vi "Get Input Index.vi"(8 "error in (no error)":errorcluster, 10 "Input Name":string, 11 "Mux in":refnum<class "Mux.lvclass">) -> (0 "error out":errorcluster, 1 "Found?":bool, 2 "Input Index":i32, 3 "Mux out":refnum<class "Mux.lvclass">)   [LabVIEW 2022 SP3]
uses:
  Mux.lvclass
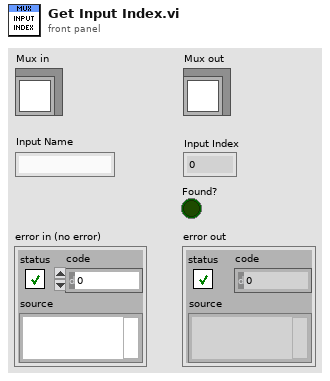
[diagram p1: front panel]
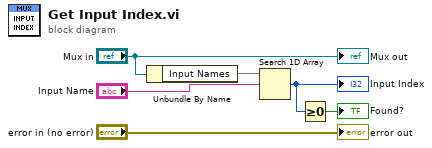
[diagram p0: block diagram]
diagram:
  n1 = Unbundle By Name("Mux in") -> ("Input Names"=w4)
  n2 = Search 1D Array(1D array=w4, element="Input Name") -> (index of element=w2:i32)  [unwired: 1 in]
  "Input Index" <- w2
  n3 = Greater Or Equal To 0?(x=w2) -> (x >= 0?=→"Found?":bool)
  "error out" <- "error in (no error)"
  "Mux out" <- "Mux in"
